vi "loop_daq.vi"(8 "error in":errorcluster, 9 "timing source":string, 11 "reference cluster":T1) -> ()   [LabVIEW 2016]
uses:
  Type Definitions/reference_cluster.ctl
  Type Definitions/vars_settings.ctl
  Type Definitions/stim_type.ctl
  Type Definitions/backlight_type.ctl
  Type Definitions/vars_runtime.ctl
  Type Definitions/data.ctl
  Type Definitions/notifier_elements_GUI.ctl
  Type Definitions/notifier_elements_DAQ.ctl
  Type Definitions/notifier_elements_write.ctl
  Type Definitions/control_references.ctl
  <vilib>/Platform/TimedLoop/XDataNode/timing_clust.ctl
  <vilib>/Platform/TimedLoop/XDataNode/nitl_modes.ctl
  <vilib>/Platform/TimedLoop/XDataNode/wakeup.ctl
  Type Definitions/tasks.ctl
  <vilib>/DAQmx/write.llb/DAQmx Write (Analog 1D DBL NChan 1Samp).vi
  <vilib>/DAQmx/miscellaneous.llb/DAQmx Fill In Error Info.vi
  <vilib>/Platform/TimedLoop/XDataNode/XDataNode.xnode
  <vilib>/Platform/TimedLoop/XDataNode/XDNodeRunTimeDep.lvlib
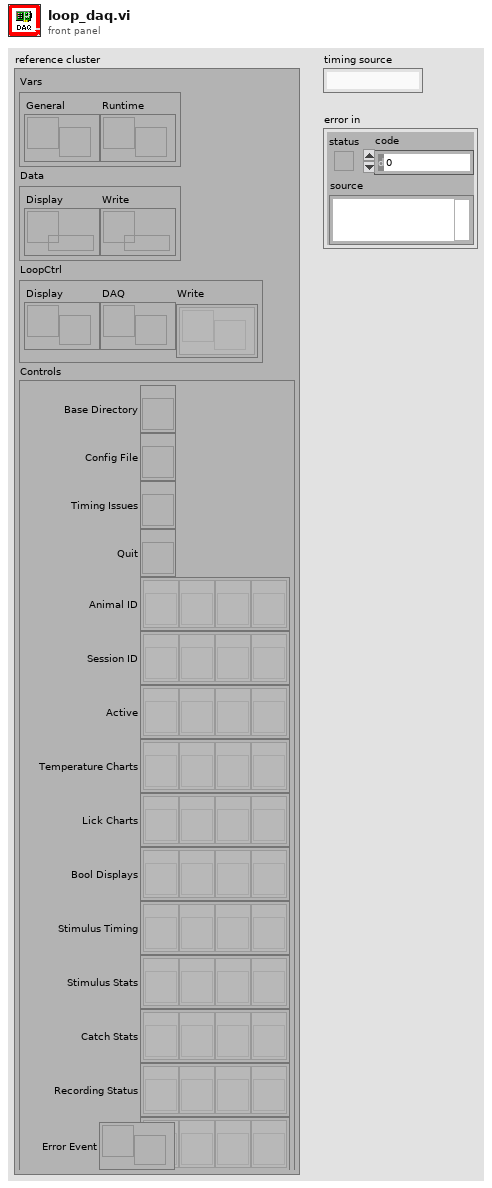
[diagram p1: front panel]
types:
  T1 = typedef "reference_cluster.ctl" = cluster{"Vars":cluster{"General":refnum<notifier>, "Runtime":refnum<notifier>}, "Data":cluster{"Display":refnum<queue>, "Write":refnum<queue>}, "LoopCtrl":cluster{"Display":refnum<notifier>, "DAQ":refnum<notifier>, "Write":refnum<notifier>[]}, "Controls":T2, "Error Event":refnum<user-event>}
  T2 = typedef "control_references.ctl" = cluster{"Base Directory":refnum<vi>, "Config File":refnum<vi>, "Timing Issues":refnum<vi>, "Quit":refnum<vi>, "Animal ID":refnum<vi>[], "Session ID":refnum<vi>[], "Active":refnum<vi>[], "Temperature Charts":refnum<vi>[], "Lick Charts":refnum<vi>[], "Bool Displays":refnum<vi>[], "Stimulus Timing":refnum<vi>[], "Stimulus Stats":refnum<vi>[], "Catch Stats":refnum<vi>[], "Recording Status":refnum<vi>[], "Pairing":refnum<vi>[]}
  T3 = typedef "XDNodeRunTimeDep.lvlib/timing_clust.ctl" = cluster{"Expected End [f-1]":u64, "Actual End [f-1]":u64, "Finished Late? [f-1]":bool, "Expected End [i-1]":u64, "Actual End [i-1]":u64, "Finished Late? [i-1]":bool, "Expected Start [i]":u64, "Actual Start [i]":u64, "Expected Start [f]":u64, "Actual Start [f]":u64, "Source Name":string, "Structure Name":string, "Period":i64, "Deadline":i64, "Offset":i64, "Start":i64, "Priority":i32, "Timeout":i32, "Mode":T4, "Wakeup Reason":T5, "Error":errorcluster, "Source Type":string, "Secondary Source Type":string, "Global End Time":u64, "Global Start Time":u64, "Frame Duration":u64, "Iteration Duration":u64, "Assigned CPU":i32, "I/O Scan Engine Mode":u32}
  T4 = typedef "XDNodeRunTimeDep.lvlib/nitl_modes.ctl" = enum32{"No Change", "Process missed periods, maintain original phase", "Discard missed periods, maintain original phase", "Process missed periods, ignore original phase", "Discard missed periods, ignore original phase"}
  T5 = typedef "XDNodeRunTimeDep.lvlib/wakeup.ctl" = enum32{"Normal", "Aborted", "Asynchronous wakeup", "Timing source error", "Timed loop error", "Timeout"}
  T6 = typedef "tasks.ctl" = cluster{"AI":refnum<k21>, "AO":refnum<k21>, "DO":refnum<k21>}
  T7 = typedef "vars_runtime.ctl" = cluster{"t wait":u16, "t stim":u16, "t square":u16, "t digStimOne":u16, "t digStimTwo":u16, "t rew":u16, "t onset":u32, "n stim":u16, "n hit":u16, "n miss":u16, "n catch":u16, "n reject":u16, "n false alarm":u16, "stim amp":sgl, "stim idx":i32, "next temp":sgl, "catch":bool, "stimulus":bool, "reward given":bool, "lick":bool, "next reward":bool, "backlight":bool, "square":bool, "digStimOne":bool, "digStimTwo":bool, "first run?":bool, "timeout":bool, "free reward":bool, "pairing":bool, "d stim":u16, "d square":u16, "n rew":u16}
  T8 = typedef "vars_settings.ctl" = cluster{"base directory":path, "data directory":path, "active":bool, "running":bool, "pairing":bool, "clean tubes":bool, "animal ID":u16, "session ID":u16, "base temp":dbl, "d wait min":u16, "d wait max":u16, "d timeout":u16, "d reward":u16, "n reward":u16, "idx stim":u16, "timeout win":u16, "lick win":i32[], "stim type":T9[], "stim dur":u16[], "stim amp":dbl[], "stim freq":u16[], "stim ramp":u16[], "stim catch":u8[], "pairing delay":i16[], "square dur":u16[], "square delay":i16[], "square freq":u8[], "square dc":u8[], "stim shape":dbl[][], "square shape":bool[][], "backlight type":T10, "backlight freq":u16, "dStimOne dur":u16[], "dStimOne delay":i16[], "dStimTwo dur":u16[], "dStimTwo delay":i16[]}
  T9 = typedef "stim_type.ctl" = enum16{"pulse", "vibration", "square", "sine"}
  T10 = typedef "backlight_type.ctl" = enum16{"none", "random", "regular"}
  T11 = typedef "notifier_elements_DAQ.ctl" = enum16{"DAQ - Initialize", "DAQ - Pause", "DAQ - Run", "DAQ - Quit"}
  T12 = cluster{"AI":refnum<k21>, "AO":refnum<k21>, "DO":refnum<k21>}
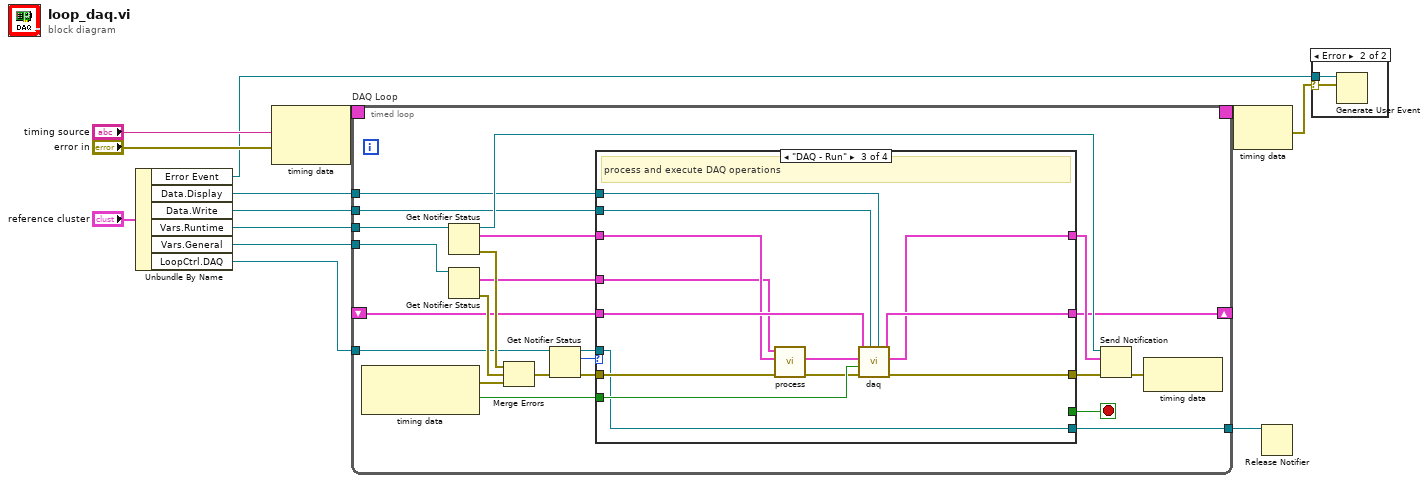
[diagram p0: block diagram]
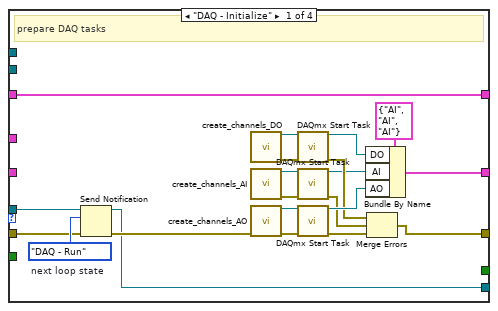
[diagram p3: hidden frame]
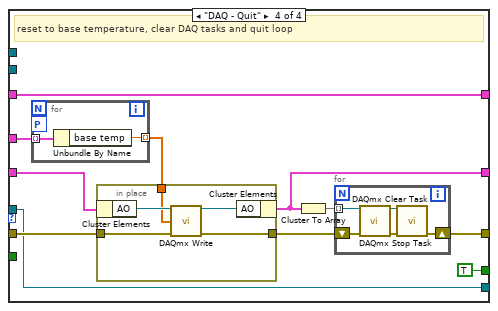
[diagram p5: hidden frame]
diagram:
  n1 = Unbundle By Name("reference cluster") -> ("Error Event"=w2:refnum<user-event>, "Data.Display"=w7:refnum<queue>, "Data.Write"=w6:refnum<queue>, "Vars.Runtime"=w5:refnum<notifier>, "Vars.General"=w4:refnum<notifier>, "LoopCtrl.DAQ"=w3:refnum<notifier>)
  n2 = node-c288("timing source", "error in") -> (w13:T3)
  n3 = timed-loop "DAQ Loop" {
    timing: w13 -> [_]
    timing-out: [_] -> w12
    shift-right: [w28] -> _
    shift-left: _ -> [w27]
    tunnel: w6 -> [w30]
    tunnel: w7 -> [w29]
    tunnel: w5 -> [w21]
    tunnel: w3 -> [w17]
    tunnel: [w14] -> w11
    tunnel: w4 -> [w22]
    stop <- w26 stop-if-true
    n4 = node-c288() -> (w18:errorcluster, w25:bool)  [unwired: 1 in]
    n5 = Get Notifier Status(notifier=w21) -> (notifier out=w36:refnum<notifier>, current notification=w20:T7[], error out=w32:errorcluster)  [unwired: 1 in, 2 out]
    n6 = Get Notifier Status(notifier=w22) -> (current notification=w19:T8[], error out=w31:errorcluster)  [unwired: 1 in, 3 out]
    n7 = Merge Errors(w32, w31, w18) -> (w33:errorcluster)
    n8 = Get Notifier Status(notifier=w17, error in (no error)=w33) -> (notifier out=w23:refnum<notifier>, current notification=w24:T11, error out=w34:errorcluster)  [unwired: 2 out]
    n9 = case shown="\"DAQ - Run\"" w24 {
      tunnel: w30 -> [_ _ w71 _]
      tunnel: w29 -> [_ _ w70 _]
      tunnel: [w53 w60 w72 w78] -> w28
      tunnel: w34 -> [w44 w58 w69 w81]
      tunnel: w27 -> [_ w60 w73 w84]
      tunnel: [w45 w58 w62 w85] -> w16
      tunnel: w25 -> [_ _ w74 _]
      tunnel: [_ _ _ TRUE] -> w26
      tunnel: w23 -> [w46 w61 w63 w76]
      tunnel: w20 -> [w37 w59 w67 w75]
      tunnel: w19 -> [_ _ w65 w80]
      tunnel: [w37 w59 w64 w75] -> w35
      tunnel: [w40 w61 w63 w76] -> w14
      frame "DAQ - Initialize" {
        w47 = notifier_elements_DAQ."DAQ - Run"  # next loop state
        # "prepare DAQ tasks"
        n10 = Send Notification(notification=w47, notifier=w46, error in (no error)=w44) -> (notifier out=w40:refnum<notifier>, error out=w43:errorcluster)
        n11 = call "create_channels_DO.vi"() -> ("task out"=w42:refnum<k21>, "error out"=w41:errorcluster)  [unwired: 14 in]
        n12 = call "create_channels_AI.vi"() -> ("task out"=w56:refnum<k21>, "error out"=w57:errorcluster)  [unwired: 14 in]
        n13 = call "create_channels_AO.vi"("error in"=w43) -> ("task out"=w38:refnum<k21>, "error out"=w39:errorcluster)  [unwired: 13 in]
        n14 = call <vilib>:"DAQmx Start Task.vi"("task/channels in"=w42, "error in"=w41) -> ("task out"=w51:refnum<k21>, "error out"=w49:errorcluster)  [unwired: 12 in]
        n15 = call <vilib>:"DAQmx Start Task.vi"("task/channels in"=w56, "error in"=w57) -> ("task out"=w48:refnum<k21>, "error out"=w50:errorcluster)  [unwired: 12 in]
        n16 = call <vilib>:"DAQmx Start Task.vi"("task/channels in"=w38, "error in"=w39) -> ("task out"=w54:refnum<k21>, "error out"=w52:errorcluster)  [unwired: 12 in]
        n17 = Bundle By Name(cluster=T6 {"AI"="AI", "AO"="AI", "DO"="AI"}, "DO"=w51, "AI"=w48, "AO"=w54) -> (w53:T6)
        n18 = Merge Errors(w49, w50, w52) -> (w45:errorcluster)
      }
      frame "DAQ - Pause" {
        # "do nothing"
      }
      frame "DAQ - Run" {
        # "process and execute DAQ operations"
        n19 = call "process.vi"("error in"=w69, "vars runtime"=w67, "vars general"=w65) -> ("error out"=w68:errorcluster, "vars runtime"=w66:T7[])  [unwired: 3 in]
        n20 = call "daq.vi"("data queue 1"=w70, "data queue 2"=w71, "error in"=w68, "finished late"=w74, "vars runtime"=w66, "task cluster"=w73) -> ("error out"=w62:errorcluster, "vars runtime"=w64:T7[], "task cluster"=w72:T12)  [unwired: 3 in]
      }
      frame "DAQ - Quit" {
        # "reset to base temperature, clear DAQ tasks and quit loop"
        n21 = for {
          tunnel: w80 -> [w92] mode=indexing
          tunnel: [w91] -> w82 mode=indexing
          workers-P: _ -> [_]
          n22 = Unbundle By Name(w92) -> ("base temp"=w91:dbl)
        }
        n23 = in-place {
          in-place-border: [w88] -> w83
          in-place-border: w81 -> [w87]
          in-place-border: w82 -> [w86]
          n24 = in-place-cluster #1(w84) -> ("AO"=w90:refnum<k21>)
          n25 = call-poly <vilib>:"DAQmx Write.vi"("task/channels in"=w90, "data"=w86, "error in"=w87) -> ("task out"=w89:refnum<k21>, "error out"=w88:errorcluster)  [unwired: 10 in, 1 out]
          n26 = in-place-cluster #1("AO"=w89) -> (w78:T6)
        }
        n27 = Cluster To Array(cluster=w78) -> (array=w79:refnum<k21>[])
        n28 = for {
          tunnel: w79 -> [w94] mode=indexing
          shift-right: [w95] -> w85
          shift-left: w83 -> [w93]
          n29 = call <vilib>:"DAQmx Stop Task.vi"("task/channels in"=w94, "error in"=w93) -> ("task out"=w97:refnum<k21>, "error out"=w96:errorcluster)  [unwired: 12 in]
          n30 = call <vilib>:"DAQmx Clear Task.vi"("task in"=w97, "error in"=w96) -> ("error out"=w95:errorcluster)  [unwired: 13 in]
        }
      }
    }
    n31 = Send Notification(notification=w35, notifier=w36, error in (no error)=w16) -> (error out=w15:errorcluster)  [unwired: 1 out]
    n32 = node-c288(w15) -> ()  [unwired: 1 out]
  }
  n33 = node-c288(w12) -> (w1:errorcluster)
  n34 = Release Notifier(notifier=w11) -> ()  [unwired: 2 in, 3 out]
  n35 = case shown="Error" w1 {
    selector: w1 -> [_ w104]
    tunnel: w2 -> [_ w105]
    frame No Error {
    }
    frame Error {
      n36 = Generate User Event(user event=w105, event data cluster=w104) -> ()  [unwired: 2 in, 2 out]
    }
  }
